vi "init.vi"(8 "error in (no error)":errorcluster, 11 "Protocol_MoveToSetpoint in":refnum<class "Protocol_MoveToSetpoint.lvclass">) -> (0 "error out":errorcluster, 3 "Protocol_MoveToSetpoint out":refnum<class "Protocol_MoveToSetpoint.lvclass">)   [LabVIEW 2011, in "Protocol_MoveToSetpoint.lvclass"]
uses:
  Protocol_MoveToSetpoint.lvclass
  protocol_Generic/Protocol_Generic.lvclass
  Protocol_MoveToSetpoint.lvclass/Protocol_MoveToSetpoint.ctl
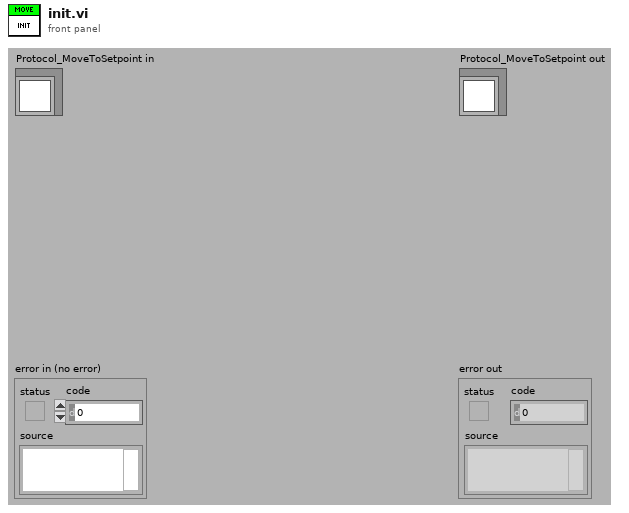
[diagram p1: front panel]
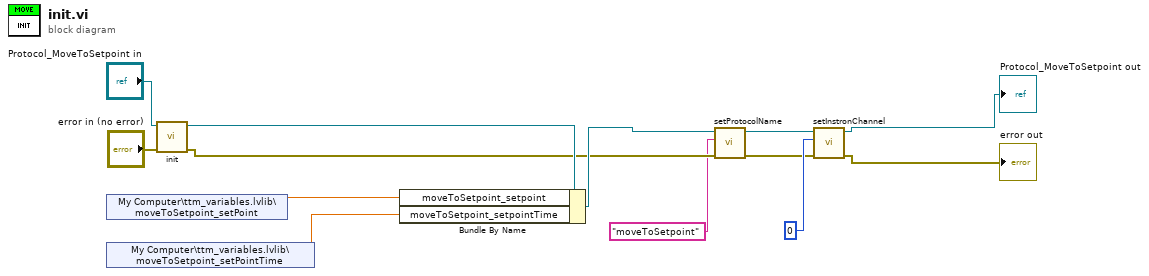
[diagram p0: block diagram]
diagram:
  n1 = shared-variable "My Computer\\ttm_variables.lvlib\\moveToSetpoint_setPoint"() -> (w10:dbl)  [unwired: 1 in, 1 out]
  n2 = shared-variable "My Computer\\ttm_variables.lvlib\\moveToSetpoint_setPointTime"() -> (w9:dbl)  [unwired: 1 in, 1 out]
  n3 = call-parent "init.vi"("error in (no error)"="error in (no error)", "Protocol_Generic in"="Protocol_MoveToSetpoint in") -> ("error out"=w3:errorcluster, "Protocol_Generic out"=w11:refnum<class "Protocol_MoveToSetpoint.lvclass">)  [unwired: 8 in]
  n4 = Bundle By Name(cluster=w11, "moveToSetpoint_setpoint"=w10, "moveToSetpoint_setpointTime"=w9) -> (w5:refnum<class "Protocol_MoveToSetpoint.lvclass">)
  n5 = call-dynamic "setProtocolName.vi"("error in (no error)"=w3, "Name"="moveToSetpoint", "Protocol_Generic in"=w5) -> ("error out"=w2:errorcluster, "Protocol_Generic out"=w4:refnum<class "Protocol_MoveToSetpoint.lvclass">)  [unwired: 7 in]
  n6 = call-dynamic "setInstronChannel.vi"("error in (no error)"=w2, "Channel"=0, "Protocol_Generic in"=w4) -> ("error out"=→"error out":errorcluster, "Protocol_Generic out"=→"Protocol_MoveToSetpoint out":refnum<class "Protocol_MoveToSetpoint.lvclass">)  [unwired: 7 in]
